vi "Download Demo.vi"(8 "error in (no error)":errorcluster, 11 "FW Path":path) -> (0 "error out":errorcluster, 3 "Success":bool)   [LabVIEW 2015, in "ST-Link.lvlib"]
uses:
  ST-Link.lvlib
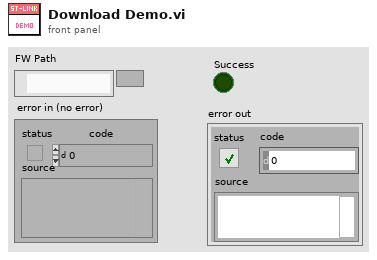
[diagram p1: front panel]
types:
  T1 = cluster{"ID":u8, "SN":string, "Protocol":enum16{"JTAG", "SWD"}, "JTAG_Freq":enum16{"9.0 MHz", "140 KHz", "281 KHz", "562 KHz", "1125 KHz", "2250 KHz", "4500 KHz"}, "SWD_Freq":enum16{"4.0 MHz", "005 KHz", "015 KHz", "025 KHz", "050 KHz", "100 KHz", "125 KHz", "240 KHz", "480 KHz", "0.9 MHz", "1.8 MHz"}, "Reset_Mode":enum16{"UR", "HOTPLUG"}, "Enable LowPower":bool}
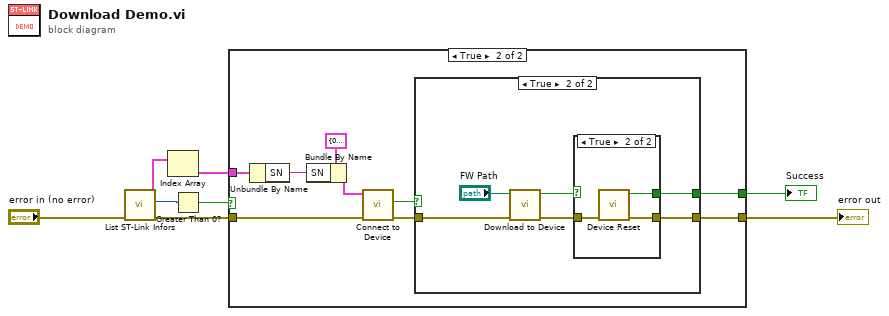
[diagram p0: block diagram]
diagram:
  n1 = call "List ST-Link Infors.vi"("error in (no error)"="error in (no error)") -> ("error out"=w4:errorcluster, "Number"=w8:i32, "ST-Links"=w6:cluster{"SN":string, "FW":string}[])  [unwired: 8 in]
  n2 = Index Array(array=w6) -> (element=w5:cluster{"SN":string, "FW":string})  [unwired: 1 in]
  n3 = Greater Than 0?(x=w8) -> (x > 0?=w7:bool)
  n4 = case shown="True" w7 {
    tunnel: w5 -> [_ w18]
    tunnel: w4 -> [w9 w14]
    tunnel: [w9 w11] -> w3
    tunnel: [_ w10] -> w1
    frame False {
    }
    frame True {
      n5 = Unbundle By Name(w18) -> ("SN"=w16:string)
      n6 = Bundle By Name(cluster=T1 {"ID"=0, "SN"="", "Protocol"=enum."SWD", "JTAG_Freq"=enum."9.0 MHz", "SWD_Freq"=enum."4.0 MHz", "Reset_Mode"=enum."UR", "Enable LowPower"=TRUE} ("Params"), "SN"=w16) -> (w15:T1)
      n7 = call "Connect to Device.vi"("error in (no error)"=w14, "Params"=w15) -> ("error out"=w12:errorcluster, "Connected OK?"=w13:bool)  [unwired: 7 in, 1 out]
      n8 = case shown="True" w13 {
        tunnel: w12 -> [w19 w25]
        tunnel: [w19 w21] -> w11
        tunnel: [_ w20] -> w10
        frame False {
        }
        frame True {
          n9 = call "Download to Device.vi"("error in (no error)"=w25, "FW Path"="FW Path") -> ("error out"=w23:errorcluster, "Download OK?"=w22:bool)  [unwired: 8 in]
          n10 = case shown="True" w22 {
            tunnel: w23 -> [w26 w29]
            tunnel: [w26 w28] -> w21
            tunnel: [_ w27] -> w20
            frame False {
            }
            frame True {
              n11 = call "Device Reset.vi"("error in (no error)"=w29) -> ("error out"=w28:errorcluster, "Reset OK?"=w27:bool)  [unwired: 9 in]
            }
          }
        }
      }
    }
  }
  "error out" <- w3
  "Success" <- w1
